vi "comm modem status flags.vi"(1 "Modem Status Flags":u32 format="%.0x") -> (0 "modem status flags cluster":T1)   [LabVIEW 2013, in "lvserial.lvlib"]
doc: "Decodes the error flags from Comm Status.vi"
uses:
  lvserial.lvlib
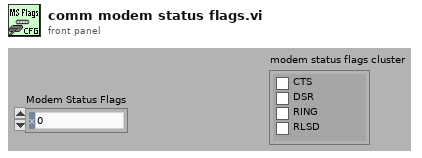
[diagram p1: front panel]
types:
  T1 = cluster{"CTS":bool, "DSR":bool, "RING":bool, "RLSD":bool}
  T2 = cluster{"Boolean array[0]":bool, "Boolean array[1]":bool, "Boolean array[2]":bool, "Boolean array[3]":bool}
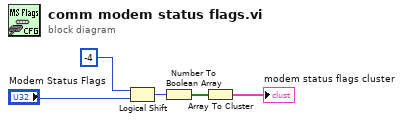
[diagram p0: block diagram]
diagram:
  n1 = Logical Shift(y=-4, x="Modem Status Flags") -> (x << y=w3:u32)
  n2 = Number To Boolean Array(number=w3) -> (Boolean array=w5:bool[])
  n3 = Array To Cluster(array=w5) -> (cluster=→"modem status flags cluster":T2)
